vi "查找首标识符.vi"(8 "offset (0)":i32 caption="偏移量(0)", 11 "XML String In":string caption="XML字符串输入") -> (0 "offset past match":i32 caption="匹配后偏移量", 1 "after tag":string caption="标识符之后", 2 "tag":string caption="标识符", 3 "before tag":string caption="标识符之前", 4 "case":enum16{"Start Tag", "Empty Element", "Content"}(ring) caption="分支", 5 "element name":string caption="元素名", 7 "node name":string caption="节点名")   [LabVIEW 2017]
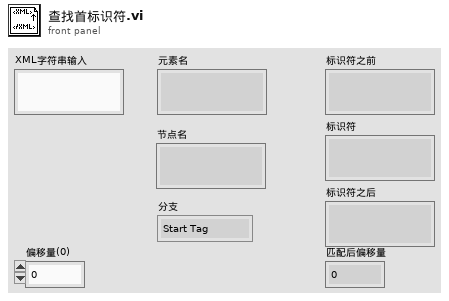
[diagram p1: front panel]
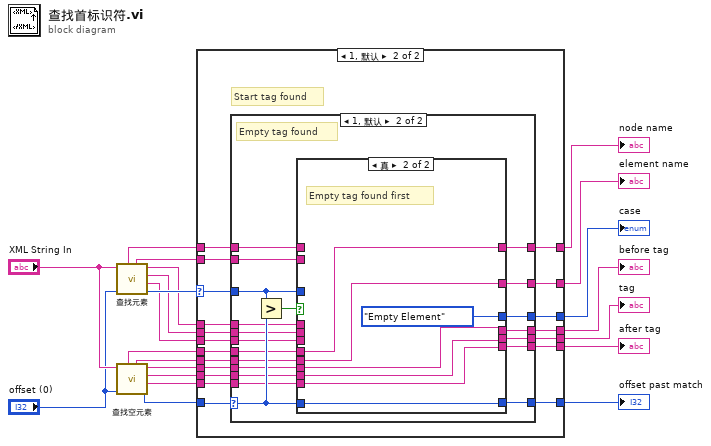
[diagram p0: block diagram]
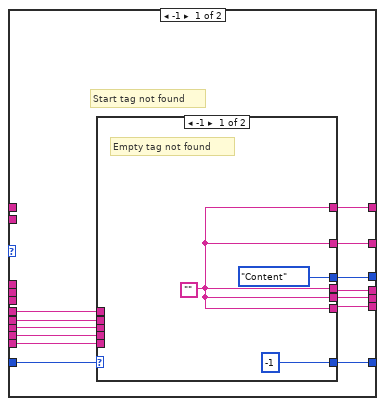
[diagram p2: hidden frame]
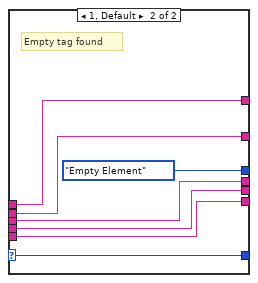
[diagram p3: hidden frame]
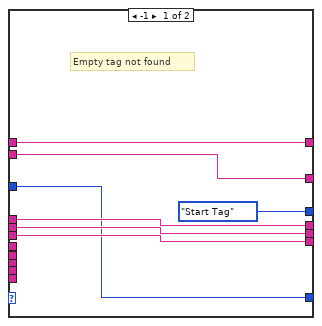
[diagram p4: hidden frame]
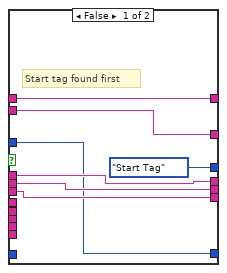
[diagram p5: hidden frame]
diagram:
  n1 = call "查找元素.vi"("offset (0)"="offset (0)", "XML String In"="XML String In") -> ("offset past match"=w19:i32, "after  tag"=w16:string, "tag"=w17:string, "before tag"=w18:string, "element name"=w9:string, "节点名"=w3:string)  [unwired: 3 in, 1 out]
  n2 = call "查找空元素.vi"("offset (0)"="offset (0)", "XML String In"="XML String In") -> ("offset past match"=w14:i32, "after  tag"=w11:string, "tag"=w12:string, "before tag"=w13:string, "element name"=w10:string, "node name"=w1:string)  [unwired: 3 in, 1 out]
  n3 = case shown="1, 默认" w19 {
    selector: w19 -> [_ w61]
    tunnel: [w33 w63] -> w4
    tunnel: w14 -> [w34 w62]
    tunnel: w13 -> [w32 w57]
    tunnel: w12 -> [w31 w56]
    tunnel: w11 -> [w30 w55]
    tunnel: w18 -> [_ w60]
    tunnel: w17 -> [_ w59]
    tunnel: w16 -> [_ w58]
    tunnel: [w29 w54] -> w21
    tunnel: [w28 w53] -> w8
    tunnel: [w27 w52] -> w20
    tunnel: w10 -> [w25 w51]
    tunnel: w9 -> [_ w50]
    tunnel: [w26 w49] -> w7
    tunnel: [w24 w48] -> w5
    tunnel: w3 -> [_ w47]
    tunnel: [w22 w46] -> w2
    tunnel: w1 -> [w23 w45]
    frame -1 {
      # "Start tag not found"
      n4 = case shown="-1" w34 {
        selector: w34 -> [_ w40]
        tunnel: [enum16{"Start Tag", "Empty Element", "Content"}."Content" enum16{"Start Tag", "Empty Element", "Content"}."Empty Element"] -> w33
        tunnel: w32 -> [_ w44]
        tunnel: w31 -> [_ w43]
        tunnel: w30 -> [_ w42]
        tunnel: [w35 w44] -> w29
        tunnel: [w35 w43] -> w28
        tunnel: [w35 w42] -> w27
        tunnel: [w35 w41] -> w26
        tunnel: w25 -> [_ w41]
        tunnel: [-1 ("offset past match") w40] -> w24
        tunnel: w23 -> [_ w38]
        tunnel: [w35 w38] -> w22
        frame -1 {
          w35 = ""
          # "Empty tag not found"
        }
        frame 1, Default {
          # "Empty tag found"
        }
      }
    }
    frame 1, Default {
      # "Start tag found"
      n5 = case shown="1, 默认" w62 {
        selector: w62 -> [_ w87]
        tunnel: [enum16{"Start Tag", "Empty Element", "Content"}."Start Tag" w90] -> w63
        tunnel: w61 -> [w66 w88]
        tunnel: w60 -> [w70 w86]
        tunnel: w59 -> [w69 w85]
        tunnel: w58 -> [w68 w84]
        tunnel: w57 -> [_ w83]
        tunnel: w56 -> [_ w82]
        tunnel: w55 -> [_ w81]
        tunnel: [w70 w80] -> w54
        tunnel: [w69 w79] -> w53
        tunnel: [w68 w78] -> w52
        tunnel: w51 -> [_ w77]
        tunnel: w50 -> [w67 w75]
        tunnel: [w67 w76] -> w49
        tunnel: [w66 w74] -> w48
        tunnel: w47 -> [w64 w73]
        tunnel: [w64 w72] -> w46
        tunnel: w45 -> [_ w71]
        frame -1 {
          # "Empty tag not found"
        }
        frame 1, Default {
          # "Empty tag found"
          n6 = Greater?(x=w88, y=w87) -> (0:w89:bool)
          n7 = case shown="真" w89 {
            tunnel: [enum16{"Start Tag", "Empty Element", "Content"}."Start Tag" enum16{"Start Tag", "Empty Element", "Content"}."Empty Element"] -> w90
            tunnel: w88 -> [w93 _]
            tunnel: w87 -> [_ w100]
            tunnel: w86 -> [w97 _]
            tunnel: w85 -> [w96 _]
            tunnel: w84 -> [w95 _]
            tunnel: w83 -> [_ w104]
            tunnel: w82 -> [_ w103]
            tunnel: w81 -> [_ w102]
            tunnel: [w97 w104] -> w80
            tunnel: [w96 w103] -> w79
            tunnel: [w95 w102] -> w78
            tunnel: w77 -> [_ w101]
            tunnel: [w94 w101] -> w76
            tunnel: w75 -> [w94 _]
            tunnel: [w93 w100] -> w74
            tunnel: w73 -> [w91 _]
            tunnel: [w91 w98] -> w72
            tunnel: w71 -> [_ w98]
            frame False {
              # "Start tag found first"
            }
            frame True {
              # "Empty tag found first"
            }
          }
        }
      }
    }
  }
  "tag" <- w8
  "before tag" <- w21
  "after tag" <- w20
  "element name" <- w7
  "offset past match" <- w5
  "case" <- w4
  "node name" <- w2
